vi "ToIPrinter.vi"(11 "OfficeTron3000":refnum<class "OfficeTron3000.lvclass">) -> (2 "OT3IPrinter":refnum<class "OT3IPrinter.lvclass">)   [LabVIEW 2018, in "OfficeTron3000.lvlib" / "OfficeTron3000.lvclass"]
uses:
  OfficeTron3000.lvclass
  OT3IPrinter/OT3IPrinter.lvclass
  OT3IPrinter/OT3IPrinter.lvclass/OT3IPrinter.ctl
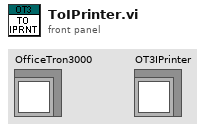
[diagram p1: front panel]
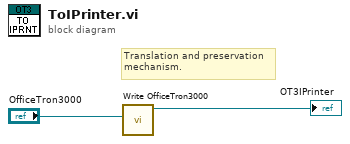
[diagram p0: block diagram]
diagram:
  # "Translation and preservation\nmechanism."
  n1 = call "Write OfficeTron3000.vi"("OfficeTron3000"="OfficeTron3000") -> ("OT3IPrinter Out"=→"OT3IPrinter":refnum<class "OT3IPrinter.lvclass">)  [unwired: 10 in]
